vi "Etalon Window.vi"(6 "Front Panel Window:Panel Bounds":T2, 7 "Üzenet be":string, 8 "Error In":errorcluster, 10 "Message":T1, 11 "Message Queue":refnum<queue>) -> (0 "Error Out":errorcluster)   [LabVIEW 2014]
uses:
  <vilib>/Utility/miscctls.llb/LVRectTypeDef.ctl
  Message.ctl
  support/Message Queue/Message Cluster.ctl
  Teszt/Teszt.ctl
  Teszt/Command.ctl
  support/Message Queue/Enqueue Message (Single).vi
  support/Message Queue/Message Queue.lvlib
panel:
  out "Üzenet":string
  in  "Hibás termék":bool
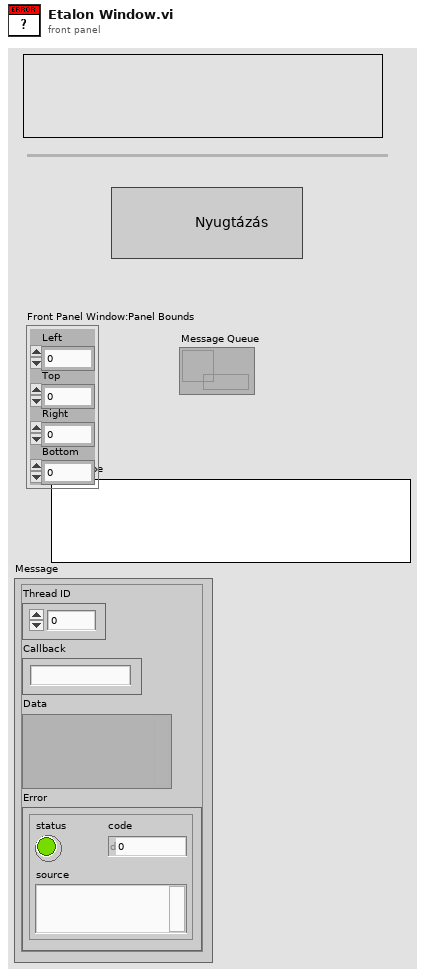
[diagram p1: front panel]
types:
  T1 = typedef "Message.ctl" = cluster{"Thread ID":u16, "Callback":string, "Data":variant, "Error":errorcluster}
  T2 = typedef "LVRectTypeDef.ctl" = cluster{"Left":i16, "Top":i16, "Right":i16, "Bottom":i16}
  T3 = typedef "Teszt.ctl" = cluster{"Thread ID":dbl, "Mérésszám":string, "Mérés/Utasítás":string, "Command":T4, "Min":string, "Max":string, "Aktív?":bool, "Log?":bool, "Kiértékelés":bool, "Etalon 1 exp":bool, "Etalon 2 exp":bool, "Etalon 3 exp":bool, "Etalon 4 exp":bool, "Etalon 5 exp":bool}
  T4 = typedef "Command.ctl" = cluster{"Parancs":string, "Paraméter 1":string, "Paraméter 2":string, "Paraméter 3":string, "Paraméter 4":string, "Paraméter 5":string, "Eredmény":string}
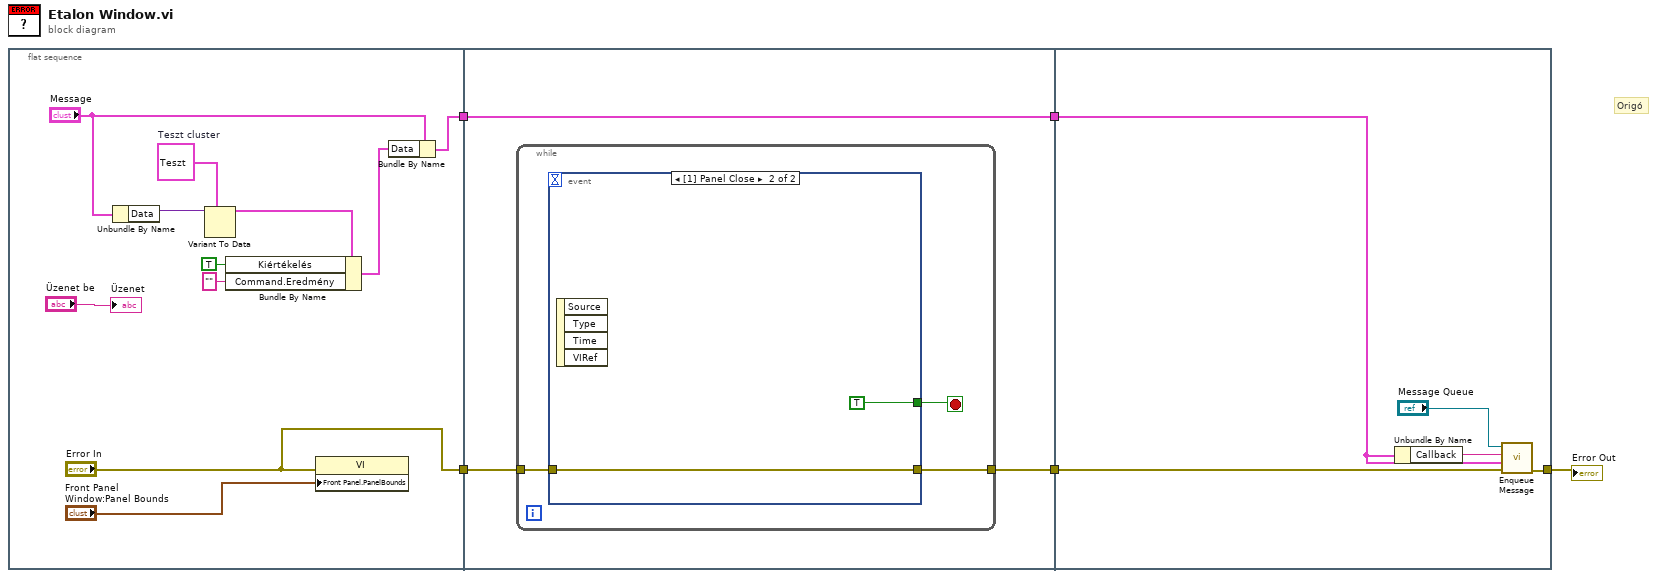
[diagram p0: block diagram]
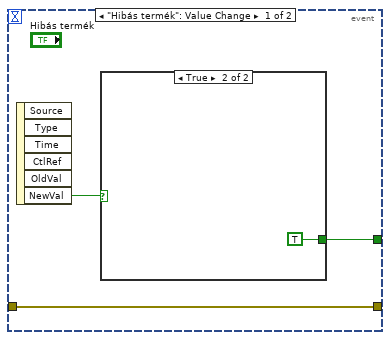
[diagram p2: hidden frame]
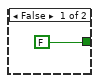
[diagram p3: hidden frame]
diagram:
  # "Origó"
  n1 = flat-sequence {
    tunnel: ["Error In"] -> w4
    tunnel: [w7] -> w2
    tunnel: w4 -> [w19]
    tunnel: [w18] -> w3
    tunnel: w2 -> [w17]
    tunnel: [w17] -> w1
    tunnel: [w33] -> w5
    tunnel: w3 -> [w34]
    tunnel: w1 -> [w31]
    frame #0 {
      w13 = T3 {"Thread ID"=0.0, "Mérésszám"="", "Mérés/Utasítás"="", "Command"={"Parancs"="", "Paraméter 1"="", "Paraméter 2"="", "Paraméter 3"="", "Paraméter 4"="", "Paraméter 5"="", "Eredmény"=""}, "Min"="", "Max"="", "Aktív?"=FALSE, "Log?"=FALSE, "Kiértékelés"=FALSE, "Etalon 1 exp"=FALSE, "Etalon 2 exp"=FALSE, "Etalon 3 exp"=FALSE, "Etalon 4 exp"=FALSE, "Etalon 5 exp"=FALSE}  # Teszt cluster
      n2 = Unbundle By Name("Message") -> ("Data"=w14:variant)
      n3 = Variant To Data(type=w13, Variant=w14) -> (data=w10:T3)  [unwired: 1 in, 1 out]
      n4 = Bundle By Name(cluster=w10, "Kiértékelés"=TRUE, "Command.Eredmény"="") -> (w9:T3)
      n5 = property on="Property Node" class="VI"(error in="Error In", "Front Panel.PanelBounds"="Front Panel Window:Panel Bounds") -> ()  [unwired: 1 in, 2 out]
      n6 = Bundle By Name(cluster="Message", "Data"=w9) -> (w7:T1)
      "Üzenet" <- "Üzenet be"
    }
    frame #1 {
      n7 = while {
        tunnel: w19 -> [w22]
        tunnel: [w21] -> w18
        stop <- w20 stop-if-true
        n8 = event shown="[1] Panel Close" {
          selector: _ -> [_ _]
          dyn-events: _ -> [_ _]
          timeout: _ -> [_ _]
          tunnel: [w25 w29] -> w21
          tunnel: w22 -> [w25 w29]
          tunnel: [w23 TRUE] -> w20
          event "Hibás termék": Value Change {
            n9 = event-data() -> ("NewVal"=w24:bool)  [unwired: 1 in, 5 out]
            n10 = case shown="True" w24 {
              tunnel: [FALSE TRUE] -> w23
              frame False {
              }
              frame True {
              }
            }
          }
          event Panel Close {
            n11 = event-data() -> ()  [unwired: 1 in, 4 out]
          }
        }
      }
    }
    frame #2 {
      n12 = Unbundle By Name(w31) -> ("Callback"=w30:string)
      n13 = call-poly "Enqueue Message.vi"("error in (no error)"=w34, "Message Data"=w31, "Message"=w30, "Message Queue"="Message Queue") -> ("error out"=w33:errorcluster)  [unwired: 6 in, 1 out]
    }
  }
  "Error Out" <- w5
